vi "cluster_v04.vi"() -> ()   [LabVIEW 2009]
panel:
  in  "Nr de perioade sinus 2":u8(knob)=2 scale=0.0..10.0
  out "XY Graph":cluster{dbl[], dbl[]}(graph)
  in  "stop":bool
  in  "Nr de perioade sinus 1":u8(knob)=8 scale=0.0..10.0
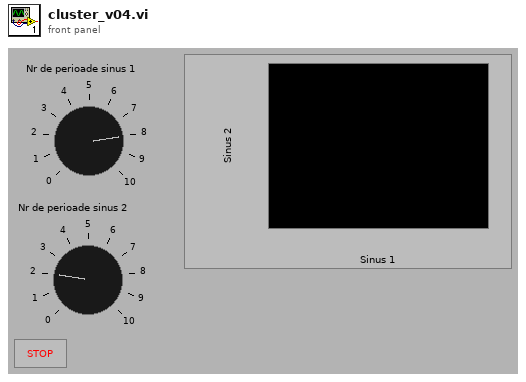
[diagram p1: front panel]
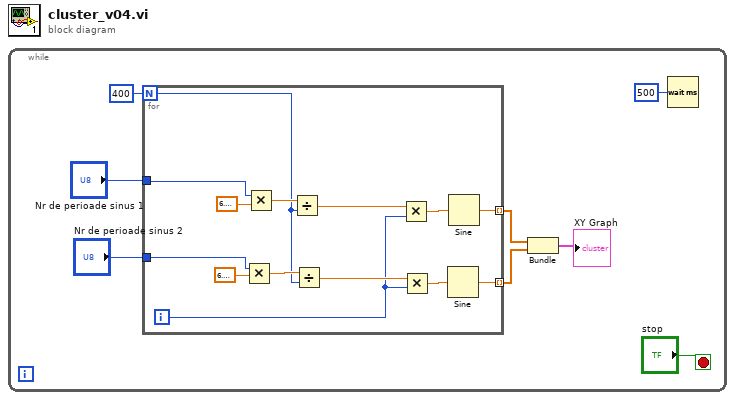
[diagram p0: block diagram]
diagram:
  n1 = while {
    stop <- "stop" stop-if-true
    n2 = for {
      N: 400 -> [w13]
      tunnel: [w22] -> w4 mode=indexing
      tunnel: "Nr de perioade sinus 1" -> [w18]
      tunnel: "Nr de perioade sinus 2" -> [w15]
      tunnel: [w10] -> w3 mode=indexing
      i -> [w9]
      n3 = Multiply(x=w15, y=6.283185307179586) -> (x*y=w14:dbl)
      n4 = Multiply(x=w18, y=6.283185307179586) -> (x*y=w19:dbl)
      n5 = Divide(x=w19, y=w13) -> (x/y=w21:dbl)
      n6 = Divide(x=w14, y=w13) -> (x/y=w12:dbl)
      n7 = Multiply(x=w21, y=w9) -> (x*y=w20:dbl)
      n8 = Multiply(x=w12, y=w9) -> (x*y=w11:dbl)
      n9 = Sine(x=w11) -> (sin(x)=w10:dbl)
      n10 = Sine(x=w20) -> (sin(x)=w22:dbl)
    }
    n11 = Bundle(w4, w3) -> (→"XY Graph":cluster{dbl[], dbl[]})  [unwired: 1 in]
    n12 = Wait (ms)(milliseconds to wait=u32 500) -> ()  [unwired: 1 out]
  }
